vi "read_PulseWidthAUX2.vi"() -> ()   [LabVIEW 2014]
panel:
  out "PulseWidth":dbl
  in  "Num Bytes to Fetch (64)":u8=64 min=1
  in  "Address (0x50)":u16=80 max=1023 format="%.0x"
  in  "Aardvark Handle":i32 min=0
  out "error out":errorcluster
  in  "error in (no error)":errorcluster
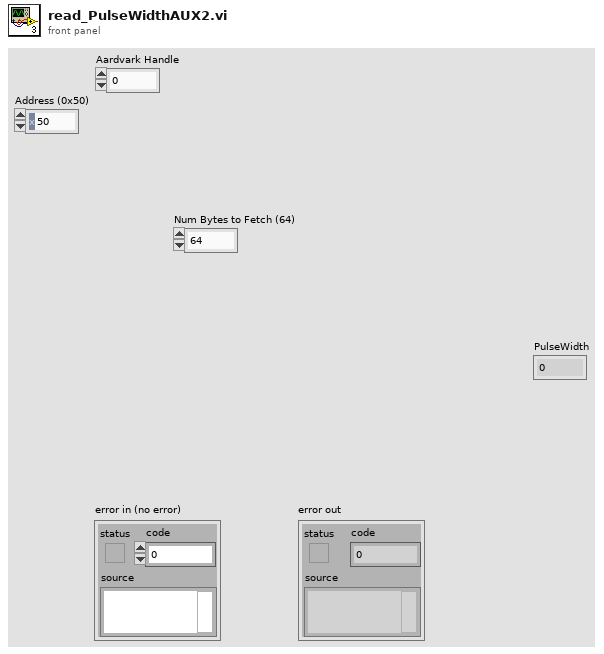
[diagram p1: front panel]
types:
  T1 = cluster{"Array[0]":u8, "Array[1]":u8, "Array[2]":u8, "Array[3]":u8, "Array[4]":u8, "Array[5]":u8, "Array[6]":u8, "Array[7]":u8, "Array[8]":u8}
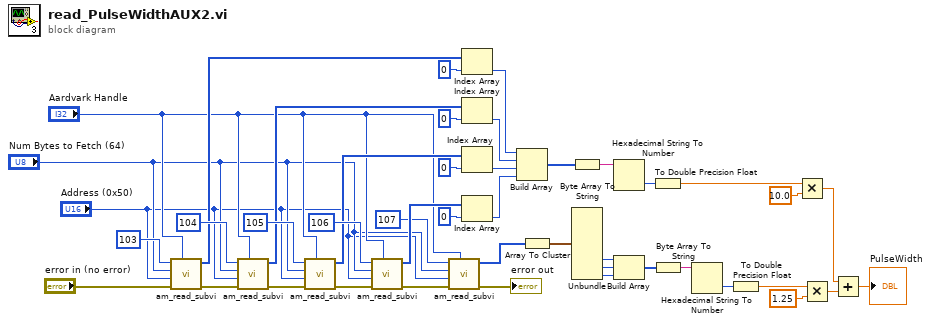
[diagram p0: block diagram]
diagram:
  n1 = call "am_read_subvi.vi"("Aardvark Handle in"="Aardvark Handle", "error in (no error)"="error in (no error)", "Address (0x50) in"="Address (0x50)", "Num Bytes to Fetch (64)"="Num Bytes to Fetch (64)", "Memory ADD"=u16 103) -> ("error out"=w43:errorcluster, "Array"=w35:u8[])  [unwired: 5 in]
  n2 = call "am_read_subvi.vi"("Aardvark Handle in"="Aardvark Handle", "error in (no error)"=w43, "Address (0x50) in"="Address (0x50)", "Num Bytes to Fetch (64)"="Num Bytes to Fetch (64)", "Memory ADD"=u16 104) -> ("error out"=w42:errorcluster, "Array"=w31:u8[])  [unwired: 5 in]
  n3 = call "am_read_subvi.vi"("Aardvark Handle in"="Aardvark Handle", "error in (no error)"=w42, "Address (0x50) in"="Address (0x50)", "Num Bytes to Fetch (64)"="Num Bytes to Fetch (64)", "Memory ADD"=u16 105) -> ("error out"=w41:errorcluster, "Array"=w30:u8[])  [unwired: 5 in]
  n4 = call "am_read_subvi.vi"("Aardvark Handle in"="Aardvark Handle", "error in (no error)"=w41, "Address (0x50) in"="Address (0x50)", "Num Bytes to Fetch (64)"="Num Bytes to Fetch (64)", "Memory ADD"=u16 106) -> ("error out"=w16:errorcluster, "Array"=w29:u8[])  [unwired: 5 in]
  n5 = call "am_read_subvi.vi"("Aardvark Handle in"="Aardvark Handle", "error in (no error)"=w16, "Address (0x50) in"="Address (0x50)", "Num Bytes to Fetch (64)"="Num Bytes to Fetch (64)", "Memory ADD"=u16 107) -> ("error out"=→"error out":errorcluster, "Array"=w13:u8[])  [unwired: 5 in]
  n6 = Index Array(array=w35, index=0) -> (element=w28:u8)
  n7 = Index Array(array=w31, index=0) -> (element=w27:u8)
  n8 = Index Array(array=w30, index=0) -> (element=w26:u8)
  n9 = Index Array(array=w29, index=0) -> (element=w25:u8)
  n10 = Build Array(w28, w27, w26, w25) -> (w23:u8[])
  n11 = Array To Cluster(array=w13) -> (cluster=w12:T1)
  n12 = Byte Array To String(unsigned byte array=w23) -> (string=w22:string)
  n13 = Unbundle(w12) -> ("Array[6]"=w9:u8, "Array[7]"=w10:u8, "Array[8]"=w11:u8)  [unwired: 6 out]
  n14 = Hexadecimal String To Number(string=w22) -> (number=w21:u32)  [unwired: 2 in, 1 out]
  n15 = Build Array(w9, w10, w11) -> (w6:u8[])
  n16 = To Double Precision Float(number=w21) -> (double precision float=w20:dbl)
  n17 = Byte Array To String(unsigned byte array=w6) -> (string=w8:string)
  n18 = Hexadecimal String To Number(string=w8) -> (number=w7:u32)  [unwired: 2 in, 1 out]
  n19 = To Double Precision Float(number=w7) -> (double precision float=w4:dbl)
  n20 = Multiply(x=w20, y=10.0) -> (x*y=w3:dbl)
  n21 = Multiply(x=w4, y=1.25) -> (x*y=w2:dbl)
  n22 = Add(x=w3, y=w2) -> (x+y=→"PulseWidth":dbl)
